vi "Main_newPower_.vi"() -> ()   [LabVIEW 2019]
uses:
  <vilib>/ptbypt/NI_PtbyPt.lvlib
panel:
  in  "Initial Motor Power":dbl
  out "error out 2":errorcluster
  out "error out 5":errorcluster
  out "error out 6":errorcluster
  in  "PID Gains":T1={"Proportional Gain (Kc)"=0.8, "Integral Gain"=0.0, "Derivative Gain"=0.0}
  in  "Reset":bool
  out "error out":errorcluster
  out "Motor 1 Correction":dbl
  out "Motor 2 Correction":dbl
  out "Motor 3 Correction":dbl
  out "Motor 4 Correction":dbl
  out "Height":dbl
  out "Filtered Correction x 2":dbl(graph)
  out "Filtered Correction y 2":dbl(graph)
  out "Filtered Correction x":dbl format="%0.2f"
  out "Filtered Correction y":dbl format="%0.2f"
  in  "low cutoff freq x":dbl=0.01 format="%#_13g"
  in  "low cutoff freq y":dbl=0.01 format="%#_13g"
  out "Raw y value":i16(graph)
  in  "Adjustment y":dbl format="%0.2f"
  in  "Adjustment x":dbl format="%0.2f"
  out "Raw x value":i16(graph)
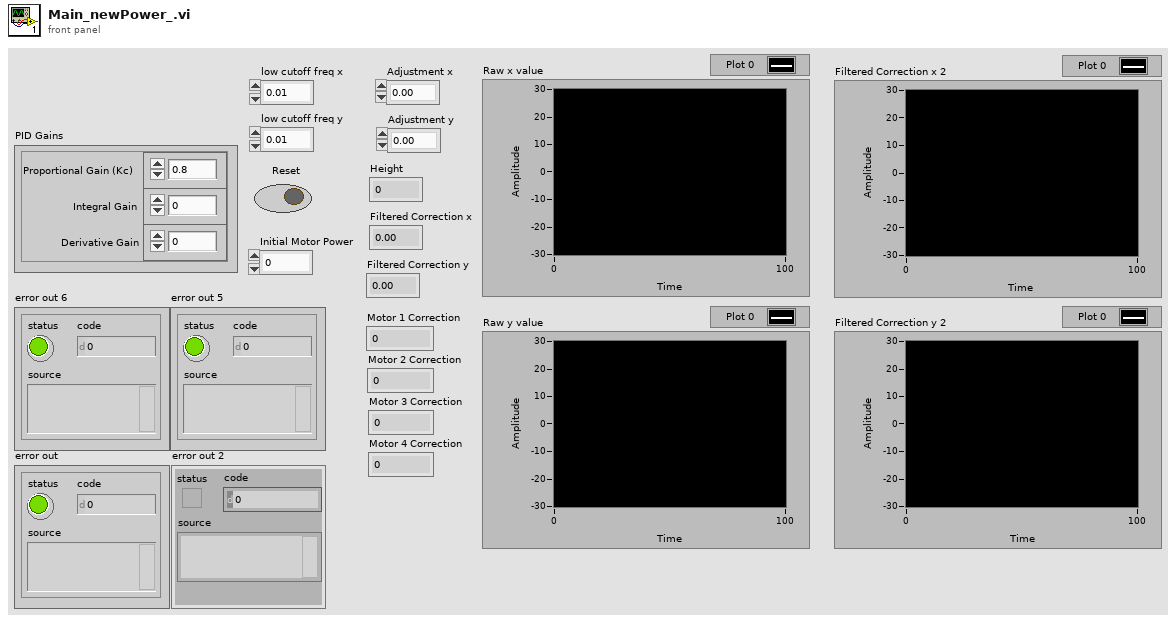
[diagram p1: front panel]
types:
  T1 = cluster{"Proportional Gain (Kc)":dbl, "Integral Gain":dbl, "Derivative Gain":dbl}
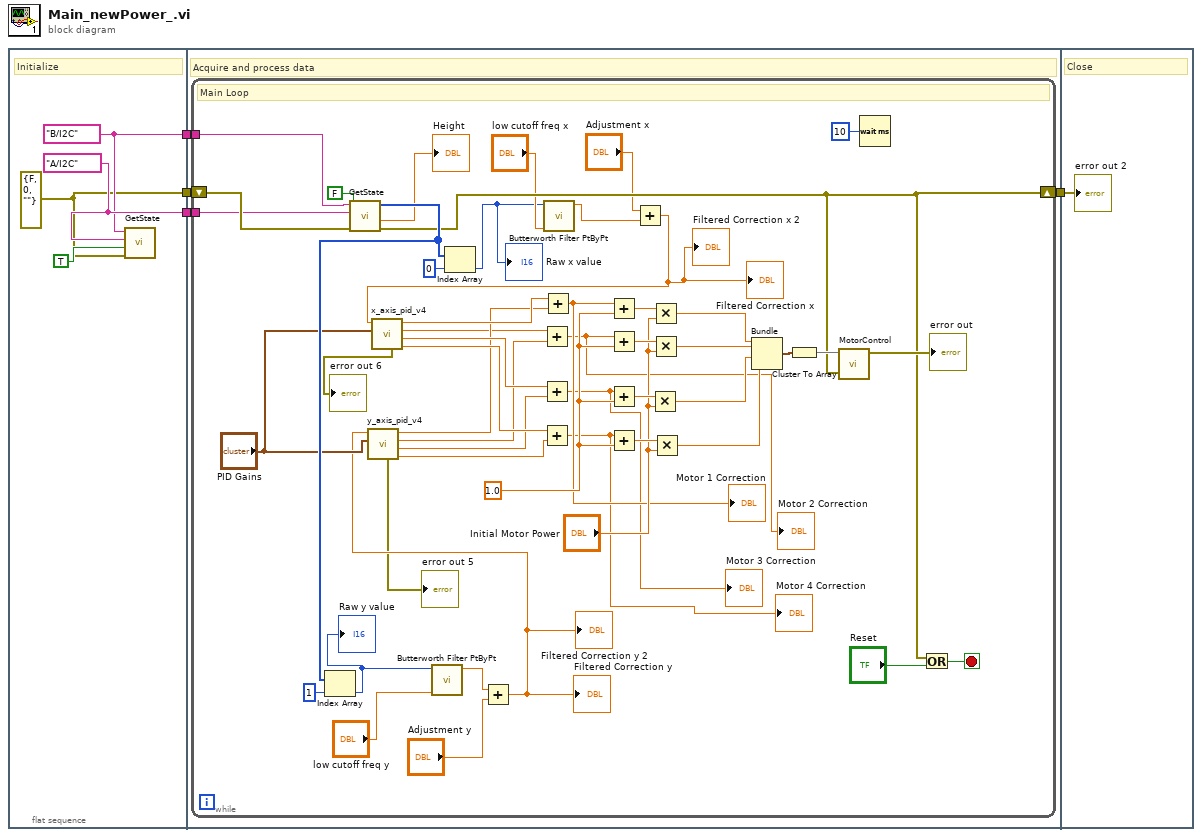
[diagram p0: block diagram]
diagram:
  n1 = flat-sequence {
    tunnel: [w7] -> w4
    tunnel: [w8] -> w3
    tunnel: [w5] -> w2
    tunnel: [w12] -> w1
    tunnel: w4 -> [w11]
    tunnel: w3 -> [w10]
    tunnel: w2 -> [w9]
    tunnel: w1 -> [w63]
    frame #0 {
      w8 = tag "A/I2C" ("IMU Channel")
      w7 = tag "B/I2C" ("LIDAR Channel")
      w5 = errorcluster {"status"=FALSE, "code"=0, "source"=""} ("error in (no error)")
      # "Initialize"
      n2 = call "GetState.vi"("error in (no error)"=w5, "Calibrate?"=TRUE, "IMU Channel"=w8, "LIDAR Channel"=w7) -> ()  [unwired: 2 in, 4 out]
    }
    frame #1 {
      # "Acquire and process data"
      n3 = while {
        shift-right: [w48] -> w12
        shift-left: w9 -> [w61]
        tunnel: w11 -> [w59]
        tunnel: w10 -> [w58]
        stop <- w62 stop-if-true
        w52 = 1.0 ("Initial Motor Power")
        # "Main Loop"
        n4 = call "GetState.vi"("error in (no error)"=w61, "Calibrate?"=FALSE, "IMU Channel"=w58, "LIDAR Channel"=w59) -> ("error out"=w48:errorcluster, "Height"=→"Height":dbl, "imu accel"=w53:i16[])  [unwired: 2 in, 1 out]
        n5 = Index Array(array=w53, index=1) -> (element=w45:i16)
        "Raw y value" <- w45
        n6 = call <vilib>:"Butterworth Filter PtByPt.vi"("low cutoff freq: fl"="low cutoff freq y", "x"=w45) -> ("Filtered x"=w44:dbl)  [unwired: 7 in, 1 out]
        n7 = Index Array(array=w53, index=0) -> (element=w40:i16)
        "Raw x value" <- w40
        n8 = Add(x=w44, y="Adjustment y") -> (x+y=w38:dbl)
        "Filtered Correction y 2" <- w38
        "Filtered Correction y" <- w38
        n9 = call "y_axis_pid_v4.vi"("PID Gains"="PID Gains", "Y In"=w38) -> ("Motor 4"=w28:dbl, "Motor 3"=w29:dbl, "Motor 2"=w30:dbl, "Motor 1"=w31:dbl, "error out"=→"error out 5":errorcluster)  [unwired: 5 in]
        n10 = call <vilib>:"Butterworth Filter PtByPt.vi"("low cutoff freq: fl"="low cutoff freq x", "x"=w40) -> ("Filtered x"=w42:dbl)  [unwired: 7 in, 1 out]
        n11 = Add(x="Adjustment x", y=w42) -> (x+y=w35:dbl)
        "Filtered Correction x 2" <- w35
        "Filtered Correction x" <- w35
        n12 = call "x_axis_pid_v4.vi"("PID Gains"="PID Gains", "X In"=w35) -> ("Motor 4"=w32:dbl, "Motor 3"=w33:dbl, "Motor 2"=w27:dbl, "Motor 1"=w34:dbl, "error out"=→"error out 6":errorcluster)  [unwired: 5 in]
        n13 = Add(x=w27, y=w30) -> (x+y=w15:dbl)
        "Motor 2 Correction" <- w15
        n14 = Add(x=w33, y=w29) -> (x+y=w14:dbl)
        "Motor 3 Correction" <- w14
        n15 = Add(x=w32, y=w28) -> (x+y=w13:dbl)
        "Motor 4 Correction" <- w13
        n16 = Add(x=w34, y=w31) -> (x+y=w16:dbl)
        "Motor 1 Correction" <- w16
        n17 = Add(x=w16, y=w52) -> (x+y=w25:dbl)
        n18 = Add(x=w15, y=w52) -> (x+y=w24:dbl)
        n19 = Add(x=w14, y=w52) -> (x+y=w23:dbl)
        n20 = Add(x=w13, y=w52) -> (x+y=w22:dbl)
        n21 = Multiply(x=w23, y="Initial Motor Power") -> (x*y=w19:dbl)
        n22 = Multiply(x=w25, y="Initial Motor Power") -> (x*y=w17:dbl)
        n23 = Multiply(x=w24, y="Initial Motor Power") -> (x*y=w18:dbl)
        n24 = Multiply(x=w22, y="Initial Motor Power") -> (x*y=w20:dbl)
        n25 = Bundle(w17, w18, w19, w20) -> (w50:cluster{dbl, dbl, dbl, dbl})  [unwired: 1 in]
        n26 = Cluster To Array(cluster=w50) -> (array=w49:dbl[])
        n27 = call "MotorControl.vi"("error in (no error)"=w48, "Array"=w49) -> ("error out"=→"error out":errorcluster)  [unwired: 9 in]
        n28 = Wait (ms)(milliseconds to wait=u32 10) -> ()  [unwired: 1 out]
        n29 = Or(x=w48, y="Reset") -> (x .or. y?=w62:bool)
      }
    }
    frame #2 {
      # "Close"
      "error out 2" <- w63
    }
  }
